vi "SCCAPI Uninitialize.vi"(8 "error in (no error)":errorcluster) -> (0 "error out":errorcluster)   [LabVIEW 2017, in "NI_SCC.lvlib"]
uses:
  <vilib>/SourceControl/sccapi/NI_SCC.lvlib
  <vilib>/SourceControl/sccapi/SCCAPI SCC Operations.ctl
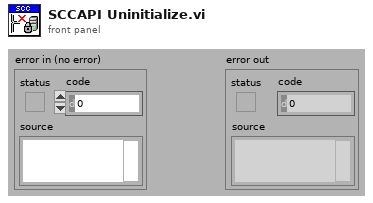
[diagram p1: front panel]
types:
  T1 = typedef "NI_SCC.lvlib/SCCAPI SCC Operations.ctl" = enum16{"Add", "Check In", "Check Out", "Close Project", "Compare Files", "Compare VIs", "Configure Project", "File History", "File Properties", "File Status", "Find All Providers", "Get Advanced Command Options", "Get File Copy", "Get Latest Version", "Get Project Name", "Get StaticVI Path", "Initialize", "Not A Source Control Reference", "Open Project", "Provider Supports Functionality", "Remove", "Run Provider", "Undo Check Out", "Uninitialize", "Is File In Local Path"}
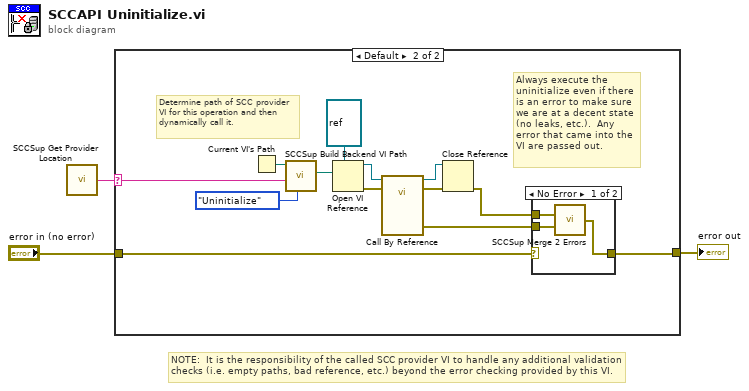
[diagram p0: block diagram]
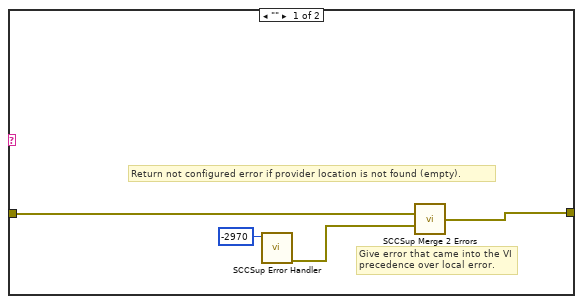
[diagram p2: hidden frame]
diagram:
  # "NOTE:  It is the responsibility of the called SCC provider VI to handle any additional validation checks (i.e. empty paths, bad reference, etc.) beyond the error checking provided by this VI."
  n1 = call <vilib>:"SCCSup Get Provider Location.vi"() -> ("provider location"=w1:string)  [unwired: 6 in]
  n2 = case shown="Default" w1 {
    selector: w1 -> [_ w8]
    tunnel: [w6 w12] -> w3
    tunnel: "error in (no error)" -> [w5 w15]
    frame "" {
      # "Give error that came into the VI precedence over local error."
      # "Return not configured error if provider location is not found (empty)."
      n3 = call <vilib>:"SCCSup Error Handler.vi"("scc error code"=-2970 ("code")) -> ("error out"=w4:errorcluster)  [unwired: 10 in]
      n4 = call <vilib>:"SCCSup Merge 2 Errors.vi"("Error IO 1"=w5, "Error IO 2"=w4) -> ("Error IO out"=w6:errorcluster)  [unwired: 13 in]
    }
    frame Default {
      # "Determine path of SCC provider VI for this operation and then dynamically call it."
      # "Always execute the uninitialize even if there is an error to make sure we are at a decent state (no leaks, etc.).  Any error that came into the VI are passed out."
      n5 = Current VI's Path() -> (path=w11:path)
      n6 = call <vilib>:"SCCSup Build Backend VI Path.vi"("scc operation"=SCCAPI_SCC_Operations."Uninitialize", "provider location"=w8, "caller path"=w11) -> ("scc backend VI path"=w10:path)  [unwired: 8 in]
      n7 = Open VI Reference(type specifier VI Refnum (for type only)=refnum<vi> refnum, vi path=w10) -> (vi reference=w19:refnum<vi>, error out=w18:errorcluster)  [unwired: 4 in]
      n8 = call-by-ref "?"(reference=w19, error in=w18) -> (reference out=w17:refnum<vi>, error out=w16:errorcluster, 0:"error out"=w13:errorcluster)  [unwired: 11 in]
      n9 = Close Reference(reference=w17, error in (no error)=w16) -> (error out=w14:errorcluster)
      n10 = case shown="No Error" w15 {
        selector: w15 -> [_ w24]
        tunnel: [w23 w24] -> w12
        tunnel: w13 -> [w21 _]
        tunnel: w14 -> [w22 _]
        frame No Error {
          n11 = call <vilib>:"SCCSup Merge 2 Errors.vi"("Error IO 1"=w22, "Error IO 2"=w21) -> ("Error IO out"=w23:errorcluster)  [unwired: 13 in]
        }
        frame Error {
        }
      }
    }
  }
  "error out" <- w3
